vi "Read deltaT.vi"(8 "error in":errorcluster, 11 "TSI 3010 in":refnum<class "TSI 3010.lvclass">) -> (0 "error out":errorcluster, 2 "deltaT":dbl, 3 "TSI 3010 out":refnum<class "TSI 3010.lvclass">)   [LabVIEW 2014, in "TSI 3010.lvclass"]
uses:
  TSI 3010.lvclass
  CPC.lvclass/CPC.ctl
  Accessors/Read Session Handle.vi
  Accessors/Write Session Handle.vi
  reusable/Session APIs/Serial/Public/Get Data/Get Double.vi
  reusable/Session APIs/Serial/Serial Session.lvclass
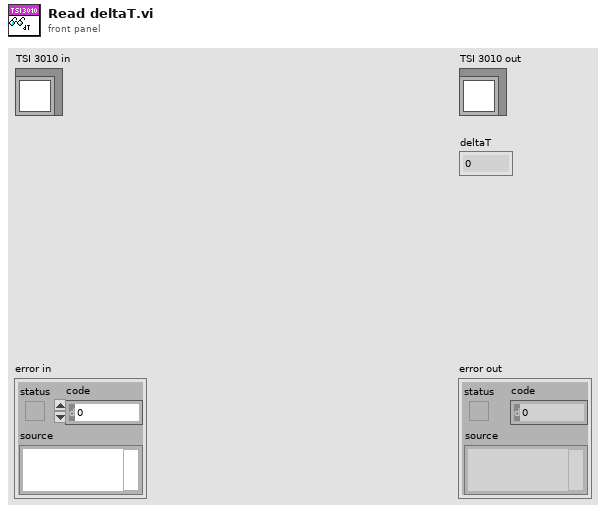
[diagram p1: front panel]
types:
  T1 = typedef "Serial Session.lvclass/Session Handle.ctl" = refnum<data-value>
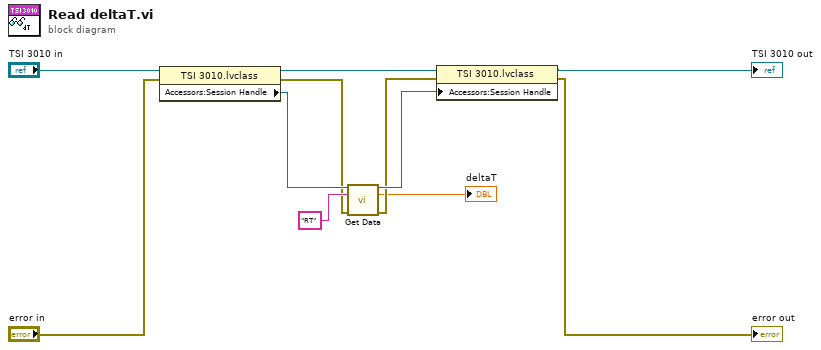
[diagram p0: block diagram]
diagram:
  n1 = property class="TSI 3010.lvclass"(reference="TSI 3010 in", error in="error in") -> (reference out=w7:refnum<class "TSI 3010.lvclass">, error out=w3:errorcluster, "Accessors:Session Handle"=w9:T1)
  n2 = call-poly "Get Data.vi"("Session Handle in"=w9, "CMD"="RT" ("string"), "error in"=w3) -> ("Session Handle out"=w8:T1, "DataOut"=→"deltaT":dbl, "error out"=w2:errorcluster)  [unwired: 10 in]
  n3 = property class="TSI 3010.lvclass"(reference=w7, error in=w2, "Accessors:Session Handle"=w8) -> (reference out=→"TSI 3010 out":refnum<class "TSI 3010.lvclass">, error out=→"error out":errorcluster)
